vi "save_conditions.vi"(0 "VI's Path":path, 2 "Load Type":string(combo), 7 "output cluster":T1, 11 "error in":errorcluster) -> (15 "error out":errorcluster)   [LabVIEW 2023]
uses:
  <vilib>/Utility/config.llb/Write Key (Double).vi
  <vilib>/Utility/config.llb/Write Key (Boolean).vi
  <vilib>/Utility/config.llb/NI_LVConfig.lvlib
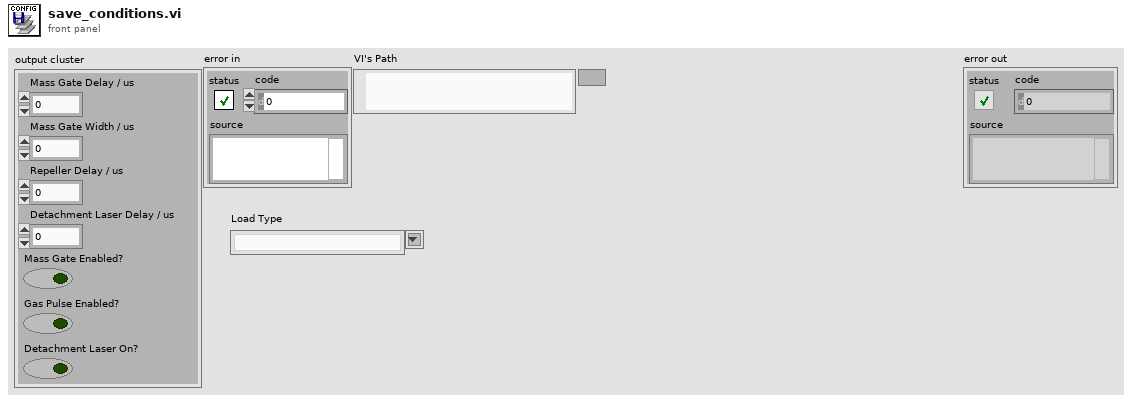
[diagram p1: front panel]
types:
  T1 = cluster{"Mass Gate Delay / us":dbl, "Mass Gate Width / us":dbl, "Repeller Delay / us":dbl, "Detachment Laser Delay / us":dbl, "Mass Gate Enabled?":bool, "Gas Pulse Enabled?":bool, "Detachment Laser On?":bool}
  T2 = typedef "NI_LVConfig.lvlib/Config Data RefNum.ctl" = refnum<k1>
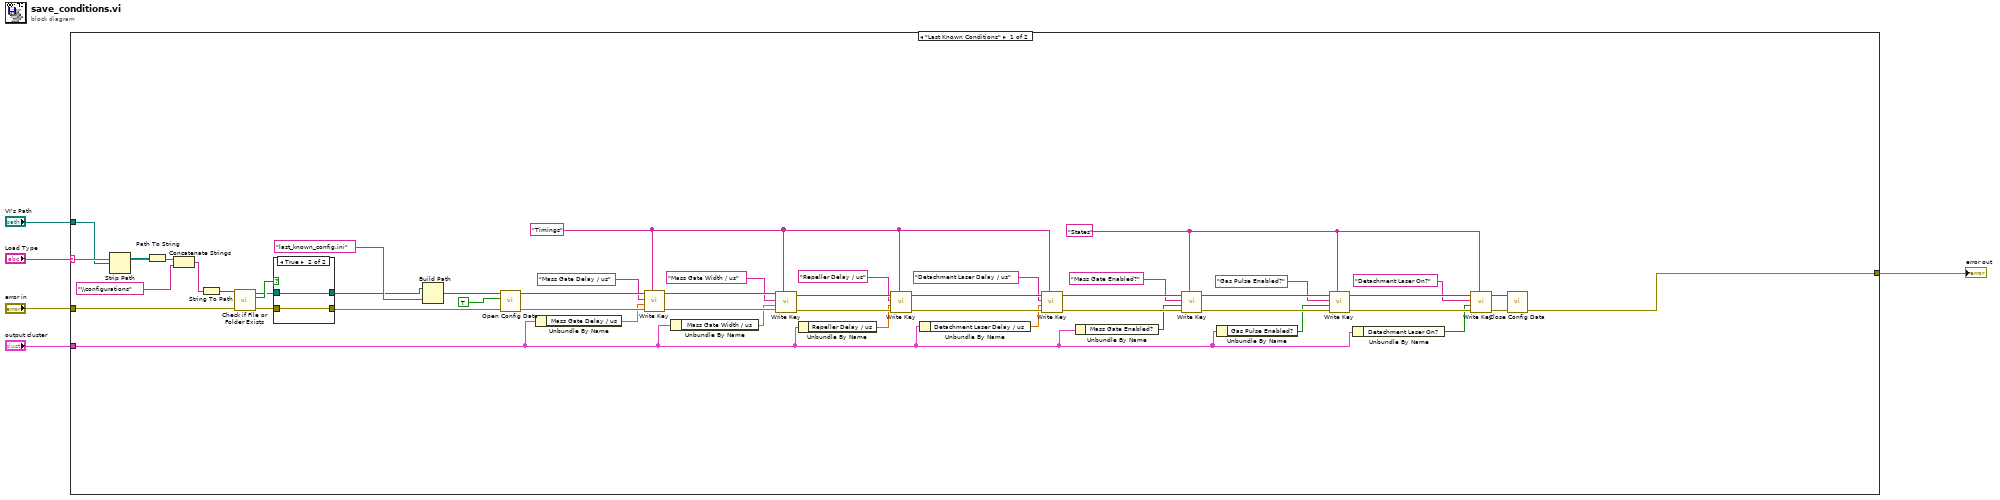
[diagram p0: block diagram]
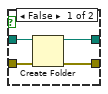
[diagram p2: hidden frame]
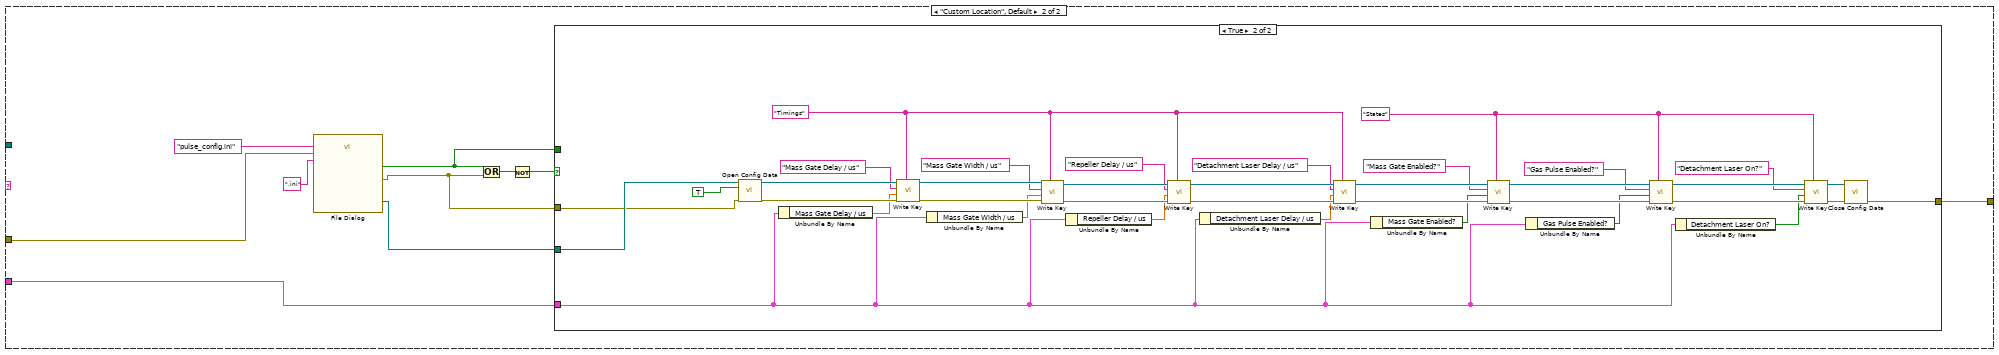
[diagram p3: hidden frame]
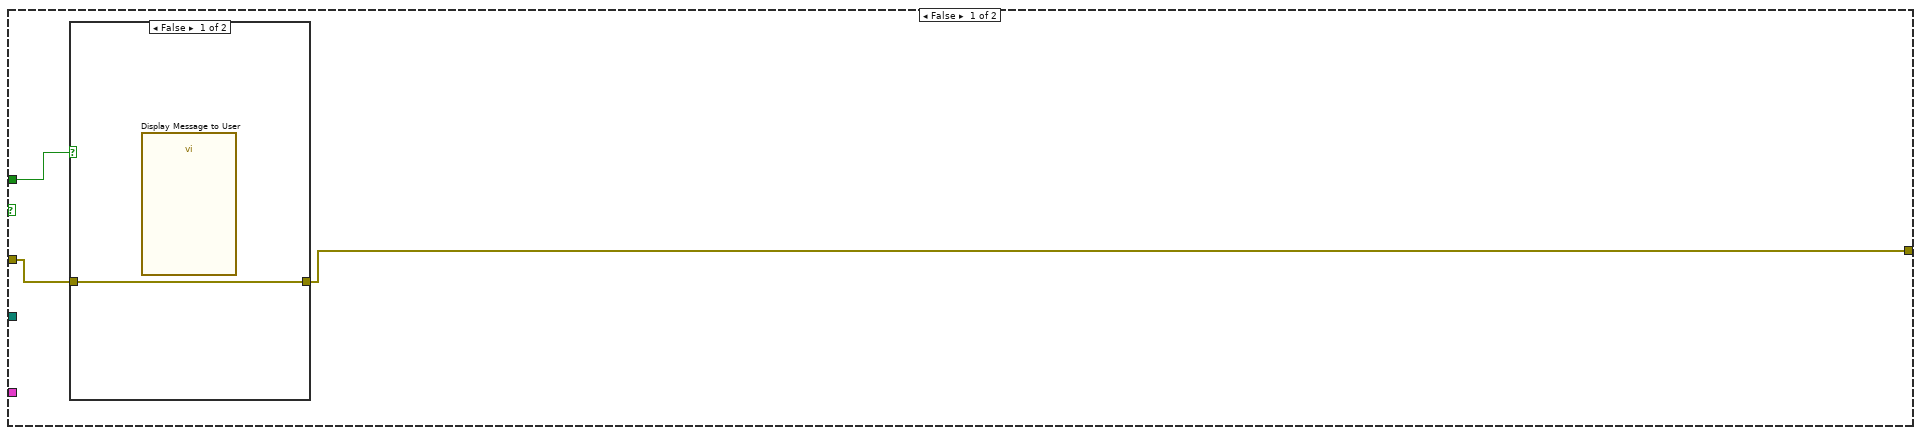
[diagram p4: hidden frame]
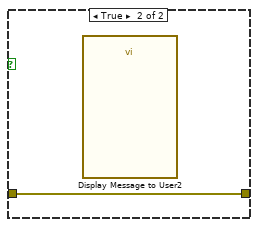
[diagram p5: hidden frame]
diagram:
  n1 = case shown="\"Last Known Conditions\"" "Load Type" {
    tunnel: [w16 w63] -> w5
    tunnel: "error in" -> [w54 w62]
    tunnel: "VI's Path" -> [w11 _]
    tunnel: "output cluster" -> [w6 w61]
    frame "Last Known Conditions" {
      w25 = "States" ("section")
      w42 = "Timings" ("section")
      n2 = Strip Path(path=w11) -> (stripped path=w15:path)  [unwired: 1 out]
      n3 = Path To String(path=w15) -> (string=w14:string)
      n4 = Concatenate Strings(w14, "\\configurations" ("string")) -> (w12:string)
      n5 = String To Path(string=w12) -> (path=w10:path)
      n6 = call <vilib>:"Check if File or Folder Exists.vi"("error in (no error)"=w54, "path"=w10) -> ("error out"=w52:errorcluster, "file or folder exists?"=w53:bool, "dup path"=w51:path)  [unwired: 7 in]
      n7 = case shown="True" w53 {
        tunnel: w52 -> [w56 w59]
        tunnel: w51 -> [w58 w60]
        tunnel: [w57 w60] -> w7
        tunnel: [w55 w59] -> w17
        frame False {
          n8 = Create Folder(path (use dialog)=w58, error in=w56) -> (created path=w57:path, error out=w55:errorcluster)  [unwired: 1 in, 1 out]
        }
        frame True {
        }
      }
      n9 = Build Path(base path=w7, name or relative path="last_known_config.ini" ("string")) -> (appended path=w8:path)
      n10 = call <vilib>:"Open Config Data.vi"("error in (no error)"=w17, "create file if necessary (T)"=TRUE, "configuration file path"=w8) -> ("error out"=w49:errorcluster, "refnum"=w50:T2)  [unwired: 6 in, 1 out]
      n11 = Unbundle By Name(w6) -> ("Mass Gate Delay / us"=w41:dbl)
      n12 = call-poly <vilib>:"Write Key.vi"("section"=w42, "error in (no error)"=w49, "value"=w41, "key"="Mass Gate Delay / us", "refnum"=w50) -> ("error out"=w47:errorcluster, "refnum out"=w48:T2)  [unwired: 4 in, 1 out]
      n13 = Unbundle By Name(w6) -> ("Mass Gate Width / us"=w40:dbl)
      n14 = call-poly <vilib>:"Write Key.vi"("section"=w42, "error in (no error)"=w47, "value"=w40, "key"="Mass Gate Width / us", "refnum"=w48) -> ("error out"=w45:errorcluster, "refnum out"=w46:T2)  [unwired: 4 in, 1 out]
      n15 = Unbundle By Name(w6) -> ("Repeller Delay / us"=w39:dbl)
      n16 = call-poly <vilib>:"Write Key.vi"("section"=w42, "error in (no error)"=w45, "value"=w39, "key"="Repeller Delay / us", "refnum"=w46) -> ("error out"=w43:errorcluster, "refnum out"=w44:T2)  [unwired: 4 in, 1 out]
      n17 = Unbundle By Name(w6) -> ("Detachment Laser Delay / us"=w38:dbl)
      n18 = call-poly <vilib>:"Write Key.vi"("section"=w42, "error in (no error)"=w43, "value"=w38, "key"="Detachment Laser Delay / us", "refnum"=w44) -> ("error out"=w32:errorcluster, "refnum out"=w33:T2)  [unwired: 4 in, 1 out]
      n19 = Unbundle By Name(w6) -> ("Mass Gate Enabled?"=w31:bool)
      n20 = call-poly <vilib>:"Write Key.vi"("section"=w25, "error in (no error)"=w32, "value"=w31, "key"="Mass Gate Enabled?", "refnum"=w33) -> ("error out"=w28:errorcluster, "refnum out"=w29:T2)  [unwired: 4 in, 1 out]
      n21 = Unbundle By Name(w6) -> ("Gas Pulse Enabled?"=w24:bool)
      n22 = call-poly <vilib>:"Write Key.vi"("section"=w25, "error in (no error)"=w28, "value"=w24, "key"="Gas Pulse Enabled?", "refnum"=w29) -> ("error out"=w26:errorcluster, "refnum out"=w27:T2)  [unwired: 4 in, 1 out]
      n23 = Unbundle By Name(w6) -> ("Detachment Laser On?"=w23:bool)
      n24 = call-poly <vilib>:"Write Key.vi"("section"=w25, "error in (no error)"=w26, "value"=w23, "key"="Detachment Laser On?", "refnum"=w27) -> ("error out"=w18:errorcluster, "refnum out"=w19:T2)  [unwired: 4 in, 1 out]
      n25 = call <vilib>:"Close Config Data.vi"("error in (no error)"=w18, "refnum"=w19) -> ("error out"=w16:errorcluster)  [unwired: 8 in, 1 out]
    }
    frame "Custom Location", Default {
      n26 = call "File Dialog"("default name"="pulse_config.ini", "error in"=w62, "pattern (all files)"=".ini") -> ("selected path"=w66:path, "cancelled"=w67:bool, "error out"=w68:errorcluster)  [unwired: 9 in, 1 out]
      n27 = Or(x=w67, y=w68) -> (x .or. y?=w70:bool)
      n28 = Not(x=w70) -> (.not. x?=w69:bool)
      n29 = case shown="True" w69 {
        tunnel: w68 -> [w72 w78]
        tunnel: w67 -> [w73 _]
        tunnel: w66 -> [_ w79]
        tunnel: [w71 w77] -> w63
        tunnel: w61 -> [_ w76]
        frame False {
          n30 = case shown="False" w73 {
            tunnel: [w74 w75] -> w71
            tunnel: w72 -> [w74 w75]
            frame False {
              n31 = call "Display Message to User"() -> ()  [unwired: 10 in, 2 out]
            }
            frame True {
              n32 = call "Display Message to User2"() -> ()  [unwired: 10 in, 2 out]
            }
          }
        }
        frame True {
          w87 = "States" ("section")
          w104 = "Timings" ("section")
          n33 = call <vilib>:"Open Config Data.vi"("error in (no error)"=w78, "create file if necessary (T)"=TRUE, "configuration file path"=w79) -> ("error out"=w111:errorcluster, "refnum"=w112:T2)  [unwired: 6 in, 1 out]
          n34 = Unbundle By Name(w76) -> ("Mass Gate Delay / us"=w103:dbl)
          n35 = call-poly <vilib>:"Write Key.vi"("section"=w104, "error in (no error)"=w111, "value"=w103, "key"="Mass Gate Delay / us", "refnum"=w112) -> ("error out"=w109:errorcluster, "refnum out"=w110:T2)  [unwired: 4 in, 1 out]
          n36 = Unbundle By Name(w76) -> ("Mass Gate Width / us"=w102:dbl)
          n37 = call-poly <vilib>:"Write Key.vi"("section"=w104, "error in (no error)"=w109, "value"=w102, "key"="Mass Gate Width / us", "refnum"=w110) -> ("error out"=w107:errorcluster, "refnum out"=w108:T2)  [unwired: 4 in, 1 out]
          n38 = Unbundle By Name(w76) -> ("Repeller Delay / us"=w101:dbl)
          n39 = call-poly <vilib>:"Write Key.vi"("section"=w104, "error in (no error)"=w107, "value"=w101, "key"="Repeller Delay / us", "refnum"=w108) -> ("error out"=w105:errorcluster, "refnum out"=w106:T2)  [unwired: 4 in, 1 out]
          n40 = Unbundle By Name(w76) -> ("Detachment Laser Delay / us"=w100:dbl)
          n41 = call-poly <vilib>:"Write Key.vi"("section"=w104, "error in (no error)"=w105, "value"=w100, "key"="Detachment Laser Delay / us", "refnum"=w106) -> ("error out"=w94:errorcluster, "refnum out"=w95:T2)  [unwired: 4 in, 1 out]
          n42 = Unbundle By Name(w76) -> ("Mass Gate Enabled?"=w93:bool)
          n43 = call-poly <vilib>:"Write Key.vi"("section"=w87, "error in (no error)"=w94, "value"=w93, "key"="Mass Gate Enabled?", "refnum"=w95) -> ("error out"=w90:errorcluster, "refnum out"=w91:T2)  [unwired: 4 in, 1 out]
          n44 = Unbundle By Name(w76) -> ("Gas Pulse Enabled?"=w86:bool)
          n45 = call-poly <vilib>:"Write Key.vi"("section"=w87, "error in (no error)"=w90, "value"=w86, "key"="Gas Pulse Enabled?", "refnum"=w91) -> ("error out"=w88:errorcluster, "refnum out"=w89:T2)  [unwired: 4 in, 1 out]
          n46 = Unbundle By Name(w76) -> ("Detachment Laser On?"=w85:bool)
          n47 = call-poly <vilib>:"Write Key.vi"("section"=w87, "error in (no error)"=w88, "value"=w85, "key"="Detachment Laser On?", "refnum"=w89) -> ("error out"=w80:errorcluster, "refnum out"=w81:T2)  [unwired: 4 in, 1 out]
          n48 = call <vilib>:"Close Config Data.vi"("error in (no error)"=w80, "refnum"=w81) -> ("error out"=w77:errorcluster)  [unwired: 8 in, 1 out]
        }
      }
    }
  }
  "error out" <- w5
